vi "A.vi"(1 "Nozzle Blockage Factor (Eq)":dbl, 2 "Nozzle Area (An)":dbl) -> (0 "Reduced Nozzle (A*)":dbl)   [LabVIEW 2017]
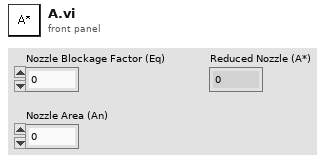
[diagram p1: front panel]
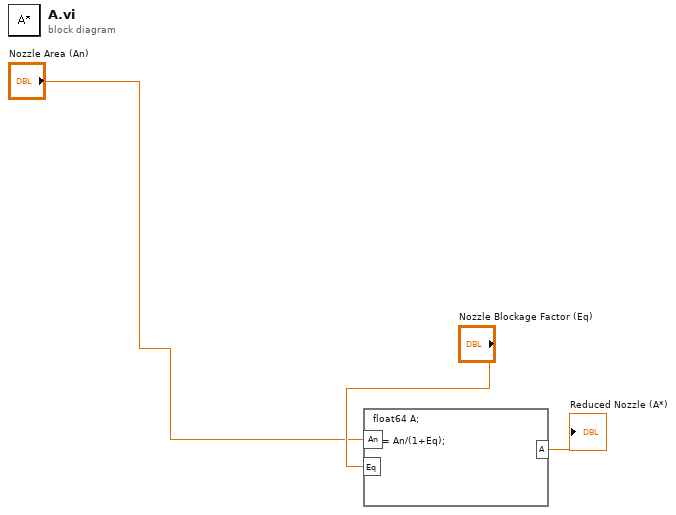
[diagram p0: block diagram]
diagram:
  n1 = formula code="float64 A;\n\nA = An/(1+Eq);"("An"="Nozzle Area (An)", "Eq"="Nozzle Blockage Factor (Eq)") -> ("A"=→"Reduced Nozzle (A*)":dbl)
